vi "Get Sessions and Channels For Pins (N Sessions).vi"(8 "error in (no error)":errorcluster, 9 "site (-1)":i32=-1, 10 "pin names":string[](array[string]), 11 "session information":T1[](array[typedef])) -> (0 "error out":errorcluster, 2 "channel list":string[][](array[string]), 3 "session indexes":i32[](array[numeric]))   [LabVIEW 2020, in "Measurement Service Helpers.lvlib"]
doc: "Gets the session index and channel list for the sessions that correspond to the given pin name input. The session index can be used to access the given session information array."
uses:
  Measurement Service Helpers.lvlib
  <vilib>/MeasurementLink/MeasurementLink Session Management Client/RPC Messages/ni_measurementlink_sessionmanagement_v1_SessionInformation.ctl
  <vilib>/MeasurementLink/MeasurementLink Session Management Client/RPC Messages/nidevice_grpc_Session.ctl
  <vilib>/MeasurementLink/MeasurementLink Session Management Client/RPC Messages/ni_measurementlink_sessionmanagement_v1_ChannelMapping.ctl
  864a66ad-3a4e-41c7-aa2d-edaf070ff137.vi
  <vilib>/Comparison/Equal/Equal Functor/Equal Functor.lvclass
  <vilib>/MeasurementLink/MeasurementLink Session Management Client/MeasurementLink Session Management Client.lvlib
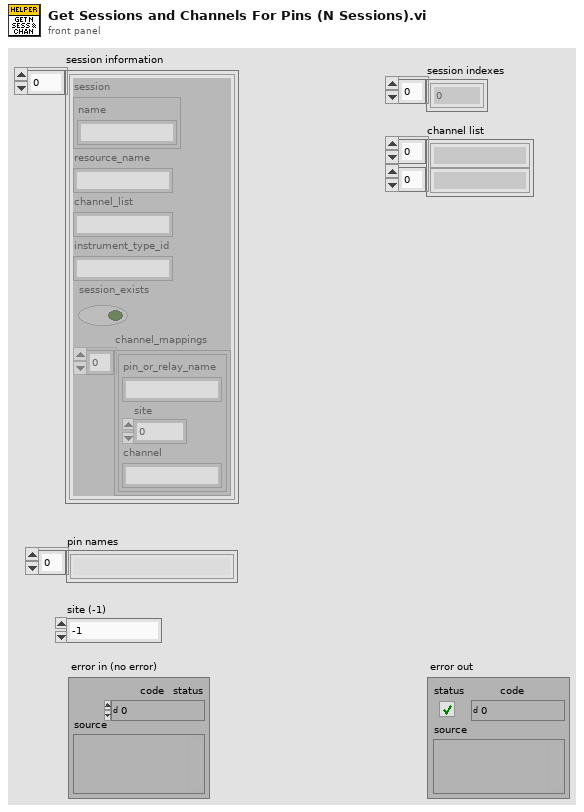
[diagram p1: front panel]
types:
  T1 = typedef "MeasurementLink Session Management Client.lvlib/ni_measurementlink_sessionmanagement_v1_SessionInformation.ctl" = cluster{"session":T2, "resource_name":string, "channel_list":string, "instrument_type_id":string, "session_exists":bool, "channel_mappings":T3[]}
  T2 = typedef "MeasurementLink Session Management Client.lvlib/nidevice_grpc_Session.ctl" = cluster{"name":string}
  T3 = typedef "MeasurementLink Session Management Client.lvlib/ni_measurementlink_sessionmanagement_v1_ChannelMapping.ctl" = cluster{"pin_or_relay_name":string, "site":i32, "channel":string}
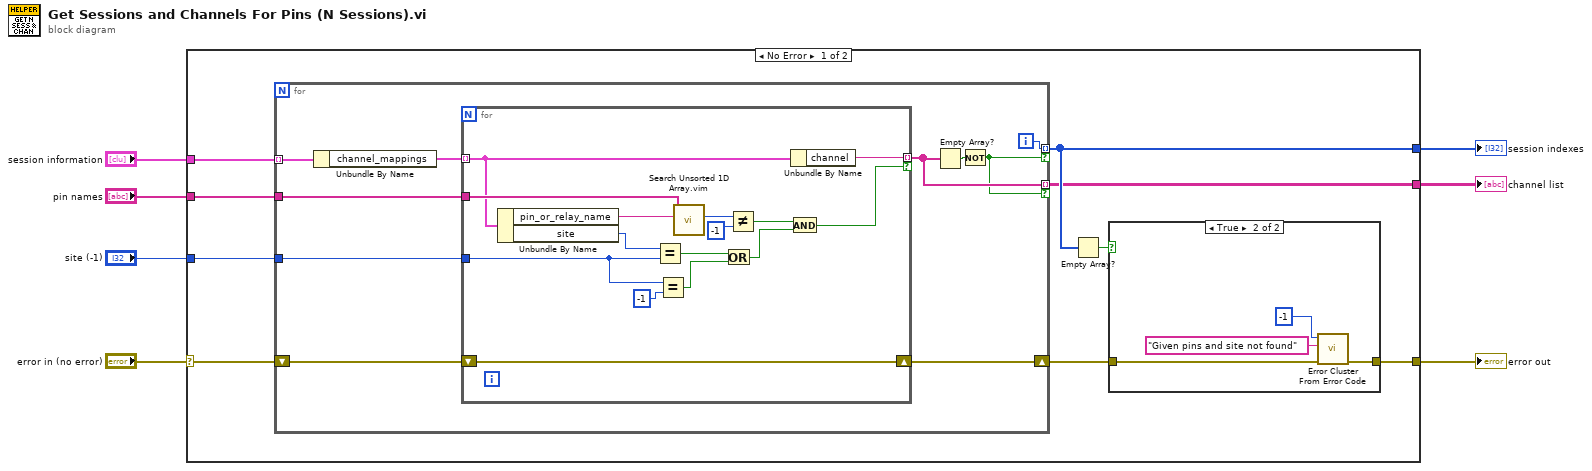
[diagram p0: block diagram]
diagram:
  n1 = case shown="No Error" "error in (no error)" {
    selector: "error in (no error)" -> [w16 w47]
    tunnel: [w11 w47] -> w6
    tunnel: "session information" -> [w14 _]
    tunnel: "pin names" -> [w13 _]
    tunnel: "site (-1)" -> [w12 _]
    tunnel: [w9 _] -> w1
    tunnel: [w8 _] -> w2
    frame No Error {
      n2 = for {
        shift-right: [w29] -> w15
        shift-left: w16 -> [w30]
        tunnel: w14 -> [w31] mode=indexing
        tunnel: w13 -> [w27]
        tunnel: w12 -> [w26]
        tunnel: [w25] -> w9 mode=indexing if=w22
        tunnel: [w24] -> w8 mode=indexing if=w22
        i -> [w25]
        n3 = Unbundle By Name(w31) -> ("channel_mappings"=w28:T3[])
        n4 = for {
          shift-right: [w46] -> w29
          shift-left: w30 -> [w46]
          tunnel: w28 -> [w40] mode=indexing
          tunnel: w27 -> [w43]
          tunnel: w26 -> [w36]
          tunnel: [w39] -> w24 mode=indexing if=w38
          n5 = Unbundle By Name(w40) -> ("pin_or_relay_name"=w41:string, "site"=w37:i32)
          n6 = Equal?(x=w37, y=w36) -> (x = y?=w33:bool)
          n7 = Equal?(x=w36, y=-1) -> (x = y?=w34:bool)
          n8 = call "Search Unsorted 1D Array.vim"("element"=w41, "unsorted 1D array"=w43) -> ("index of element"=w45:i32)  [unwired: 9 in]
          n9 = Or(x=w33, y=w34) -> (x .or. y?=w32:bool)
          n10 = Not Equal?(x=w45, y=-1) -> (x != y?=w42:bool)
          n11 = And(x=w42, y=w32) -> (x .and. y?=w38:bool)
          n12 = Unbundle By Name(w40) -> ("channel"=w39:string)
        }
        n13 = Empty Array?(array=w24) -> (empty?=w23:bool)
        n14 = Not(x=w23) -> (.not. x?=w22:bool)
      }
      n15 = Empty Array?(array=w9) -> (empty?=w10:bool)
      n16 = case shown="True" w10 {
        tunnel: w15 -> [w17 w21]
        tunnel: [w17 w20] -> w11
        frame False {
        }
        frame True {
          n17 = call <vilib>:"Error Cluster From Error Code.vi"("error in (no error)"=w21, "error message (\"\")"="Given pins and site not found" ("error message (\"\")"), "error code (0)"=-1) -> ("error out"=w20:errorcluster)  [unwired: 6 in]
        }
      }
    }
    frame Error {
    }
  }
  "error out" <- w6
  "channel list" <- w2
  "session indexes" <- w1
